vi "RealtimeDNITrack.vi"() -> ()   [LabVIEW 2017]
uses:
  <extravilib>/ChannelInstances/Tag-bool.lvlib
  <vilib>/platform/TimedLoop/XDataNode/XDataNode.xnode
  <vilib>/Platform/TimedLoop/XDataNode/nitl_modes.ctl
  <vilib>/Platform/TimedLoop/XDataNode/XDNodeRunTimeDep.lvlib
  <vilib>/Platform/TimedLoop/XDataNode/wakeup.ctl
  <vilib>/Platform/TimedLoop/XDataNode/timing_clust.ctl
  <vilib>/daq.io/MQTT LabVIEW Client/MQTT_Functions.lvlib
  <vilib>/daq.io/MQTT LabVIEW Client/Controls/MessageType.ctl
  <vilib>/daq.io/MQTT LabVIEW Client/Controls/Retain_Flag.ctl
  <vilib>/daq.io/MQTT LabVIEW Client/Controls/DUP_Flag.ctl
  <vilib>/daq.io/MQTT LabVIEW Client/Controls/QoS.ctl
  C:/Users/Labview/Downloads/Two Loops Ap/Two Loops Ap/Channel Scan Functional Global Op.ctl
  <vilib>/daq.io/MQTT LabVIEW Client/Controls/Connect_Flags.ctl
  <vilib>/daq.io/MQTT LabVIEW Client/Controls/Connection_Return_Codes.ctl
panel:
  in  "Tab Control":T1(tab)
  out "Corrected Phi":string
  out "Corrected Theta":string
  out "Current Time":string
  out "Corrected DNI":dbl
  in  "Working Directory":path=path "G:/Chad/Tracking Software/Analysis/LabVIEW-Outdoor-Tracking-App"
  out "Time of tracking start":string
  out "Sunset":string
  out "Sunrise":string
  in  "stop":bool
  in  "Stop Reading":bool
  out "standard error 3":string
  out "return code 3":i32
  in  "Script 3":string="solar_system.py"
  out "standard error":string
  out "return code":i32
  in  "error in (no error)":errorcluster
  in  "Sample Frequency (minutes)":string="1"
  out "Seconds to wait\nfor next minute":dbl
  in  "Script":string="cos_correct_v2.py"
  in  "Script 2":string="angle_to_position.py"
  out "standard error 2":string
  out "return code 2":i32
  out "Time":string
  out "Current Y":dbl
  out "Cos Corrected DNI":cluster{dbl[], dbl[]}(graph)
  out "Tracking":cluster{"X Coords":dbl[], "Y Coords":dbl[]}[](graph)
  out "Current X":dbl
  in  "Show full history":bool
  out "Waveform Graph":dbl[][](graph)
  in  "X Length":i32
  in  "Client ID":string="LVSubscribeClient"
  in  "Connect Flags":T2
  out "Granted QoS Levels":T3[](array[typedef])
  in  "Subscription Info Array":cluster{"Topic":string, "QoS":T3}[](array[cluster])=[{"Topic"="testtopic/LVMQTT", "QoS"=enum."At most once"}]
  in  "MQTT Broker":cluster{"address (IP)":string, "port":u16}={"address (IP)"="broker.hivemq.com", "port"=1883}
  out "Connection Status":T4=enum."Connection refused: Server unavailable"
  out "Messages":T6(array[cluster])
  out "MQTT Feed":string
  in  "Ping period (ms)":u32
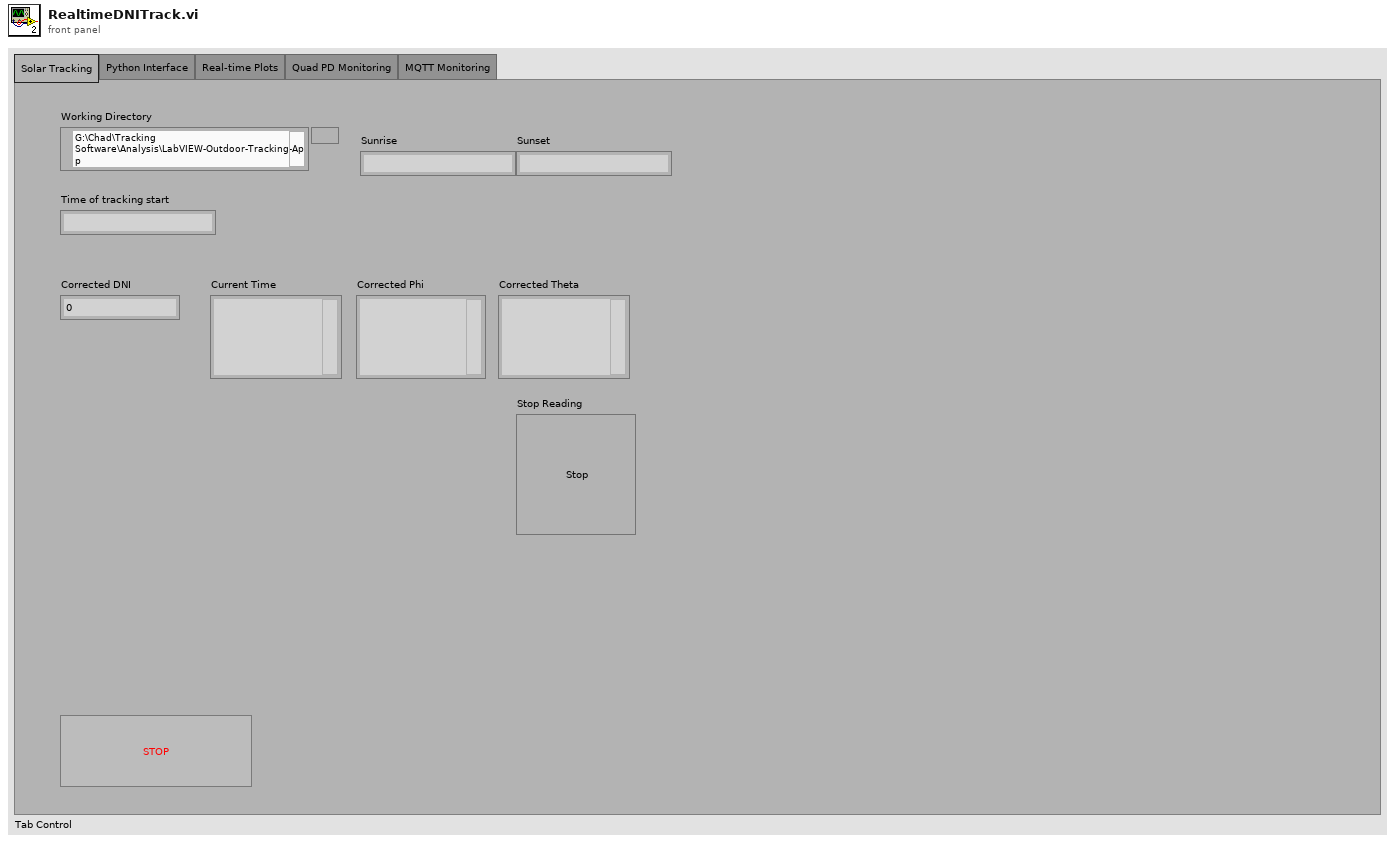
[diagram p1: front panel]
types:
  T1 = enum32{"Solar Tracking", "Python Interface", "Real-time Plots", "Quad PD Monitoring", "MQTT Monitoring"}
  T2 = typedef "MQTT_Functions.lvlib/Connect_Flags.ctl" = cluster{"user name":bool, "password":bool, "will retain":bool, "will flag":bool, "clean session":bool, "reserved":bool, "will QoS":T3}
  T3 = typedef "MQTT_Functions.lvlib/QoS.ctl" = enum8{"At most once", "At least once", "Exactly once", "Reserved"}
  T4 = typedef "MQTT_Functions.lvlib/Connection_Return_Codes.ctl" = enum16{"Connection accepted", "Connection refused: unacceptable protocol version", "Connection refused: identifier rejected", "Connection refused: Server unavailable", "Connection refused: bad user name or password", "Connection refused: not authorized"}
  T5 = typedef "MQTT_Functions.lvlib/MessageType.ctl" = enum32{"Reserved", "CONNECT", "CONNACK", "PUBLISH", "PUBACK", "PUBREC", "PUBREL", "PUBCOMP", "SUBSCRIBE", "SUBACK", "UNSUBSCRIBE", "UNSUBACK", "PINGREQ", "PINGRESP", "DISCONNECT", "Reserved2"}
  T6 = cluster{"Message ID":u16, "Topic Name":string, "Message ":string, "MessageType":T5}[]
  T7 = typedef "XDNodeRunTimeDep.lvlib/timing_clust.ctl" = cluster{"Expected End [f-1]":u64, "Actual End [f-1]":u64, "Finished Late? [f-1]":bool, "Expected End [i-1]":u64, "Actual End [i-1]":u64, "Finished Late? [i-1]":bool, "Expected Start [i]":u64, "Actual Start [i]":u64, "Expected Start [f]":u64, "Actual Start [f]":u64, "Source Name":string, "Structure Name":string, "Period":i64, "Deadline":i64, "Offset":i64, "Start":i64, "Priority":i32, "Timeout":i32, "Mode":T8, "Wakeup Reason":T9, "Error":errorcluster, "Source Type":string, "Secondary Source Type":string, "Global End Time":u64, "Global Start Time":u64, "Frame Duration":u64, "Iteration Duration":u64, "Assigned CPU":i32, "I/O Scan Engine Mode":u32}
  T8 = typedef "XDNodeRunTimeDep.lvlib/nitl_modes.ctl" = enum32{"No Change", "Process missed periods, maintain original phase", "Discard missed periods, maintain original phase", "Process missed periods, ignore original phase", "Discard missed periods, ignore original phase"}
  T9 = typedef "XDNodeRunTimeDep.lvlib/wakeup.ctl" = enum32{"Normal", "Aborted", "Asynchronous wakeup", "Timing source error", "Timed loop error", "Timeout"}
  T10 = typedef "MQTT_Functions.lvlib/DUP_Flag.ctl" = bool
  T11 = typedef "MQTT_Functions.lvlib/Retain_Flag.ctl" = bool
  T12 = cluster{"QoS":T3, "DUP":T10, "Retain":T11, "Keep Alive (sec)":u16}
  T13 = enum16{"None", "On Hover", "On Key Focus", "On Hover or Key Focus"}
  T14 = typedef "Channel Scan Functional Global Op.ctl" = enum16{"Init", "Insert Value", "Get Values"}
  T15 = cluster{"Message ID":u16, "Topic Name":string, "Message":string, "MessageType":T5}[]
  T16 = cluster{cluster{"X Coords":dbl[], "Y Coords":dbl[]}, cluster{dbl[], dbl[]}, cluster{dbl[], dbl[]}}
  T17 = cluster{"Message ID":u16, "Topic Name":string, "Message":string, "MessageType":T5}
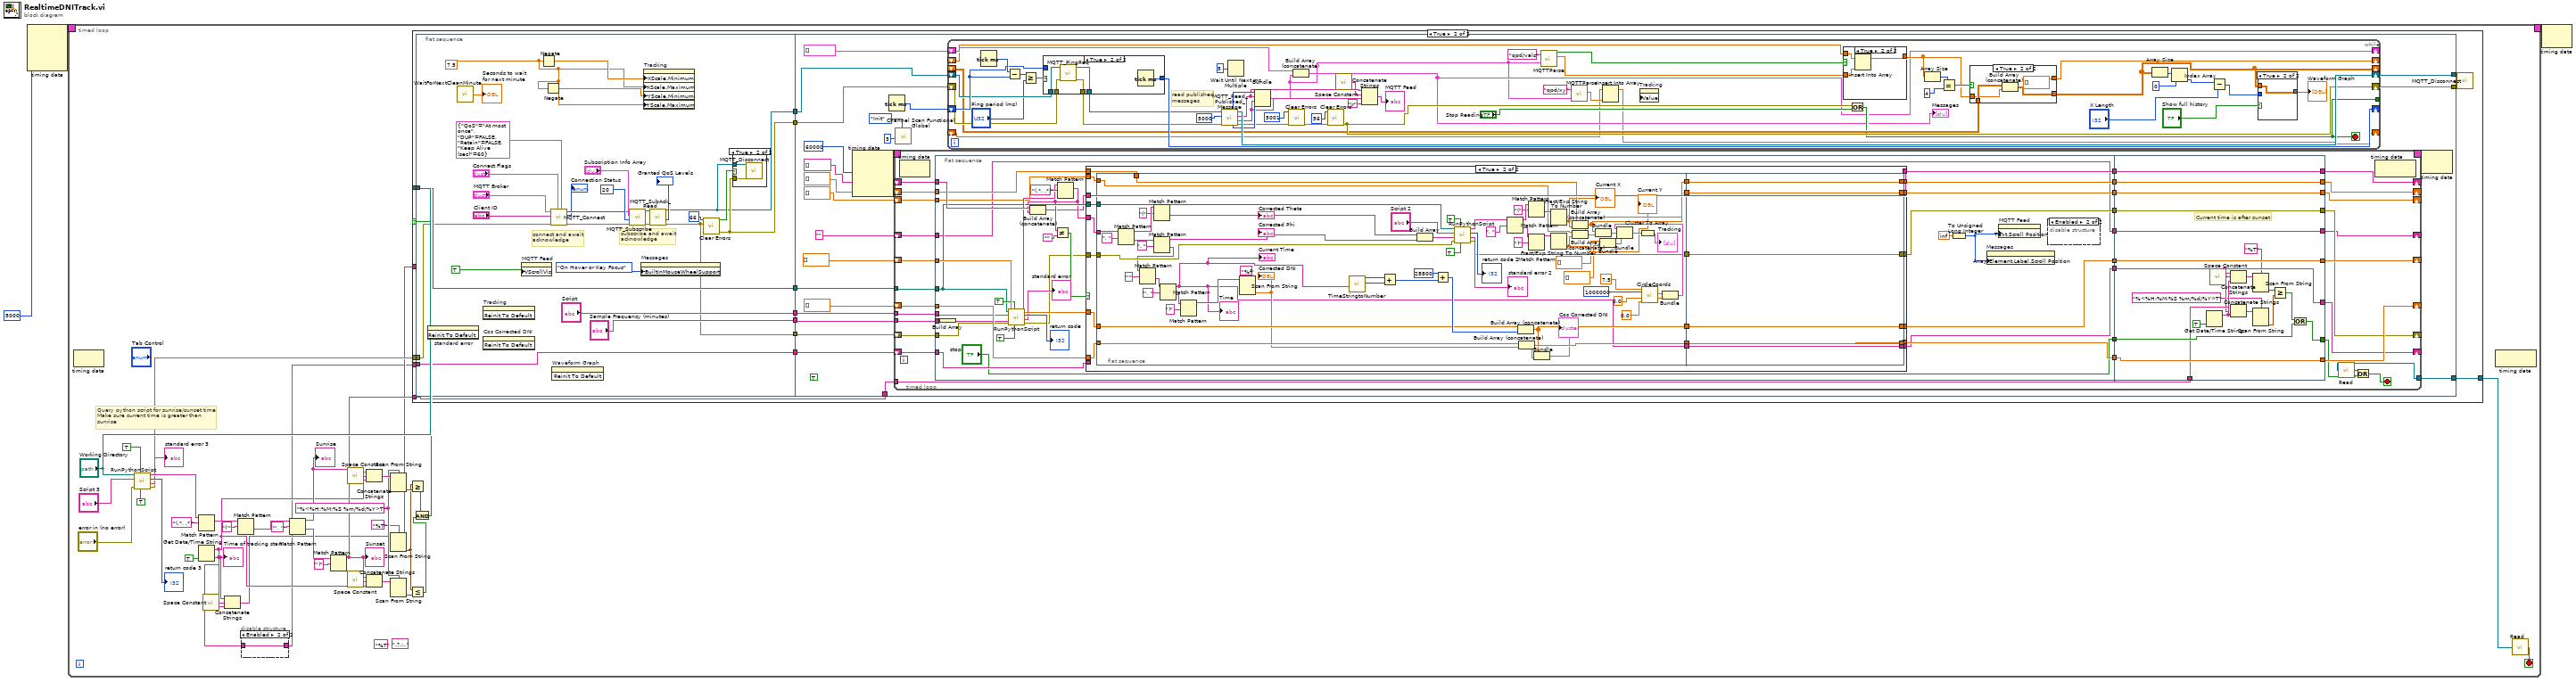
[diagram p0: block diagram]
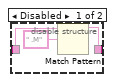
[diagram p2: hidden frame]
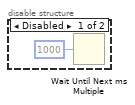
[diagram p5: hidden frame]
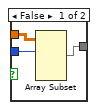
[diagram p7: hidden frame]
diagram:
  n1 = node-c288(i64 5000 ("Period")) -> (w3:T7)  [unwired: 3 in]
  n2 = timed-loop {
    timing: w3 -> [_]
    timing-out: [_] -> w2
    stop <- w41 stop-if-true
    w8 = "%<%H:%M:%S %m/%d/%Y>T" ("format string")
    (unwired) "%T" ("format string")
    (unwired) ".?.:.." ("regular expression")
    # "Query python script for sunrise/sunset time\nMake sure current time is greater than\nsunrise"
    n3 = node-c288() -> ()  [unwired: 1 in, 1 out]
    n4 = call "RunPythonScript.vi"("Run minimized? (F)"=TRUE, "Wait until completion? (T)"=TRUE, "error in (no error)"="error in (no error)", "Script"="Script 3", "Script Directory"="Working Directory") -> ("error out"=w23:errorcluster, "standard error"=→"standard error 3":string, "return code"=→"return code 3":i32, "standard output"=w37:string)  [unwired: 3 in]
    n5 = Match Pattern(string=w37, regular expression="(.*, .*)") -> (match substring=w36:string)  [unwired: 1 in, 3 out]
    n6 = Get Date/Time String(want seconds? (F)=TRUE) -> (date string=w14:string, time string=w5:string)  [unwired: 2 in]
    "Time of tracking start" <- w5
    n7 = call <vilib>:"Space Constant.vi"() -> ("String"=w22:string)
    n8 = Concatenate Strings(w5, w22, w14) -> (w6:string)
    n9 = Match Pattern(string=w36, regular expression="('") -> (after substring=w32:string)  [unwired: 1 in, 3 out]
    n10 = disable-structure shown="Enabled" {
      disable-tunnel: w5 -> [w44 w45]
      disable-tunnel: [w42 w45] -> w4
      frame Disabled {
        n11 = Match Pattern(string=w44, regular expression=" .M") -> (before substring=w42:string)  [unwired: 1 in, 3 out]
      }
      frame Enabled {
      }
    }
    n12 = Match Pattern(string=w32, regular expression="', '") -> (before substring=w19:string, after substring=w31:string)  [unwired: 1 in, 2 out]
    "Sunrise" <- w19
    n13 = Match Pattern(string=w31, regular expression="')") -> (before substring=w15:string)  [unwired: 1 in, 3 out]
    "Sunset" <- w15
    n14 = call <vilib>:"Space Constant.vi"() -> ("String"=w21:string)
    n15 = call <vilib>:"Space Constant.vi"() -> ("String"=w17:string)
    n16 = Concatenate Strings(w19, w21, w14) -> (w20:string)
    n17 = Concatenate Strings(w15, w17, w14) -> (w16:string)
    n18 = Scan From String(format string=w8, input string=w20) -> (output 1=w24:timestamp)  [unwired: 3 in, 3 out]
    n19 = Scan From String(format string="%T", input string=w6) -> (output 1=w18:timestamp)  [unwired: 3 in, 3 out]
    n20 = Scan From String(format string=w8, input string=w16) -> (output 1=w13:timestamp)  [unwired: 3 in, 3 out]
    n21 = Greater Or Equal?(x=w18, y=w24) -> (x >= y?=w12:bool)
    n22 = Less Or Equal?(x=w18, y=w13) -> (x <= y?=w11:bool)
    n23 = And(x=w12, y=w11) -> (x .and. y?=w10:bool)
    n24 = case shown="True" w10 {
      tunnel: "Working Directory" -> [_ w55]
      tunnel: w23 -> [_ w54]
      tunnel: w15 -> [_ w52]
      tunnel: [_ w53] -> w9
      tunnel: w6 -> [_ _]
      tunnel: w4 -> [_ w50]
      frame False {
      }
      frame True {
        n25 = flat-sequence {
          tunnel: [w64] -> w56
          tunnel: ["Script"] -> w57
          tunnel: [w82] -> w58
          tunnel: ["Sample Frequency (minutes)"] -> w59
          tunnel: w55 -> [w82]
          tunnel: w54 -> [w81]
          tunnel: w50 -> [w78]
          tunnel: [w78] -> w51
          tunnel: [w61] -> w49
          tunnel: [w60] -> w46
          tunnel: w59 -> [w106]
          tunnel: w58 -> [w107]
          tunnel: w57 -> [w108]
          tunnel: w56 -> [w102]
          tunnel: [w95] -> w53
          tunnel: w52 -> [w104]
          tunnel: w51 -> [w103]
          tunnel: w49 -> [w98]
          tunnel: [w96] -> w48
          tunnel: [w99] -> w47
          tunnel: w46 -> [w97]
          frame #0 {
            w85 = 7.5
            # "connect and await\nacknowledge"
            # "subscribe and await\nacknowledge"
            n26 = invoke on="standard error" class="Str" method="Reinit To Default"() -> ()  [unwired: 3 in, 3 out]
            n27 = call "WaitForNextCleanMinute.vi"() -> ("Seconds to wait"=→"Seconds to wait\nfor next minute":dbl)  [unwired: 1 in]
            n28 = invoke on="Tracking" class="XYGraph (strict)" method="Reinit To Default"() -> ()  [unwired: 3 in, 3 out]
            n29 = invoke on="Cos Corrected DNI" class="XYGraph (strict)" method="Reinit To Default"() -> ()  [unwired: 3 in, 3 out]
            n30 = property on="MQTT Feed" class="Str"("VScrollVis"=TRUE ("Vertical Scrollbar Visible")) -> ()  [unwired: 2 in, 2 out]
            n31 = Negate(x=w85) -> (-x=w87:dbl)
            n32 = Negate(x=w85) -> (-x=w86:dbl)
            n33 = call <vilib>:"MQTT_Connect.vi"("Connect Meta"=T12 {"QoS"=enum."At most once", "DUP"=FALSE, "Retain"=FALSE, "Keep Alive (sec)"=60}, "Client ID"="Client ID", "Connect Flags"="Connect Flags", "error in (no error)"=w81, "MQTT Broker"="MQTT Broker") -> ("error out"=w66:errorcluster, "Connection Status"=→"Connection Status":T4, "connection ID out"=w68:refnum<k5>)  [unwired: 4 in]
            n34 = invoke on="Waveform Graph" class="WFGraph (strict)" method="Reinit To Default"() -> ()  [unwired: 3 in, 3 out]
            n35 = call <vilib>:"MQTT_Subscribe.vi"("error in (no error)"=w66, "Message ID"=u16 20, "Subscription Info Array"="Subscription Info Array", "connection ID"=w68) -> ("error out"=w72:errorcluster, "connection ID out"=w73:refnum<k5>)  [unwired: 6 in]
            n36 = property on="Messages" class="Arr (strict)"("BuiltInMouseWheelSupport"=T13."On Hover or Key Focus" ("Built-In Mouse Wheel Support")) -> ()  [unwired: 2 in, 2 out]
            n37 = property on="Tracking" class="XYGraph (strict)"("XScale.Minimum"=w87, "XScale.Maximum"=w85, "YScale.Minimum"=w86, "YScale.Maximum"=w85) -> ()  [unwired: 2 in, 2 out]
            n38 = call <vilib>:"MQTT_SubAck_Read.vi"("error in (no error)"=w72, "connection ID"=w73) -> ("error out"=w64:errorcluster, "Granted QoS Levels"=→"Granted QoS Levels":T3[], "connection ID out"=w60:refnum<k5>)  [unwired: 7 in]
            n39 = call <vilib>:"Clear Errors.vi"("error in (no error)"=w64, "specific error code to clear (0: all)"=66) -> ("error out"=w61:errorcluster, "specific error cleared?"=w62:bool)  [unwired: 4 in]
            n40 = case shown="True" w62 {
              tunnel: w60 -> [_ w89]
              tunnel: w61 -> [_ w88]
              frame False {
              }
              frame True {
                n41 = call <vilib>:"MQTT_Disconnect.vi"("error in (no error)"=w88, "connection ID"=w89) -> ()  [unwired: 9 in, 1 out]
              }
            }
          }
          frame #1 {
            (unwired) TRUE ("Key Focus")
            n42 = node-c288(i64 60000 ("Period")) -> (w94:T7)  [unwired: 3 in]
            n43 = Tick Count (ms)() -> (millisecond timer value=w100:u32)
            n44 = timed-loop {
              tunnel: w106 -> [w141]
              shift-right: [w145] -> _
              shift-left: dbl[] [] -> [w146]
              shift-right: [w144] -> _
              shift-left: dbl[] [] -> [w142]
              shift-right: [w134] -> _
              shift-left: string[] [] -> [w143]
              tunnel: w107 -> [w135]
              tunnel: w108 -> [w140]
              shift-right: [w138] -> _
              shift-left: dbl[] [] -> [w137]
              shift-right: [w136] -> _
              shift-left: dbl[] [] -> [w139]
              shift-right: [w126] -> _
              shift-left: w103 -> [w125]
              tunnel: w104 -> [w124]
              tunnel: [w117] -> w95
              shift-right: [w121] -> _
              shift-left: "" -> [w120]
              shift-right: [w123] -> _
              shift-left: w102 -> [w119]
              timing: w94 -> [_]
              timing-out: [_] -> w93
              stop <- w114 stop-if-true
              n45 = node-c288() -> ()  [unwired: 1 in, 1 out]
              n46 = flat-sequence {
                tunnel: w146 -> [w180]
                tunnel: w143 -> [w177]
                tunnel: w142 -> [w176]
                tunnel: w119 -> [w175]
                tunnel: w141 -> [w170]
                tunnel: w140 -> [w168]
                tunnel: w139 -> [w167]
                tunnel: w137 -> [w165]
                tunnel: w135 -> [w163]
                tunnel: [w179] -> w133
                tunnel: [w178] -> w132
                tunnel: [w166] -> w131
                tunnel: ["stop"] -> w130
                tunnel: [w164] -> w129
                tunnel: [w150] -> w128
                tunnel: [w157] -> w127
                tunnel: w125 -> [w156]
                tunnel: [w151] -> w122
                tunnel: w120 -> [w149]
                tunnel: [w149] -> w118
                tunnel: [w296] -> w134
                tunnel: [w297] -> w136
                tunnel: [w298] -> w138
                tunnel: [w299] -> w144
                tunnel: [w300] -> w145
                tunnel: w133 -> [w300]
                tunnel: w132 -> [w299]
                tunnel: w131 -> [w298]
                tunnel: w130 -> [w295]
                tunnel: w129 -> [w297]
                tunnel: w128 -> [w296]
                tunnel: w127 -> [w290]
                tunnel: [w290] -> w126
                tunnel: w124 -> [w288]
                tunnel: [w283] -> w116
                tunnel: [w282] -> w123
                tunnel: w122 -> [w282]
                tunnel: [w281] -> w121
                tunnel: w118 -> [w281]
                frame #0 {
                  n47 = Build Array(w170) -> (w169:string[])
                  n48 = call "RunPythonScript.vi"("Run minimized? (F)"=TRUE ("run minimized? (F)"), "Wait until completion? (T)"=TRUE ("wait until completion? (T)"), "error in (no error)"=w175, "Array of arguments to script"=w169, "Script"=w168, "Script Directory"=w163) -> ("error out"=w152:errorcluster, "standard error"=→"standard error":string, "return code"=→"return code":i32, "standard output"=w172:string)  [unwired: 2 in]
                  n49 = Match Pattern(string=w172, regular expression="(.*, .*)") -> (match substring=w160:string)  [unwired: 1 in, 3 out]
                  n50 = Build Array (concatenate)(w177, w160) -> (w158:string[])
                  n51 = Not Equal?(x=w160, y="") -> (x != y?=w159:bool)
                  n52 = case shown="True" w159 {
                    tunnel: w180 -> [w186 w209]
                    tunnel: [w186 w208] -> w179
                    tunnel: [w187 w207] -> w178
                    tunnel: w176 -> [w187 w206]
                    tunnel: w167 -> [w189 w205]
                    tunnel: [w188 w204] -> w166
                    tunnel: w165 -> [w188 w203]
                    tunnel: [w189 w202] -> w164
                    tunnel: w163 -> [_ w201]
                    tunnel: w160 -> [_ w198]
                    tunnel: [w185 w190] -> w150
                    tunnel: w158 -> [w185 w190]
                    tunnel: [w184 w197] -> w157
                    tunnel: w156 -> [w184 _]
                    tunnel: w152 -> [w183 w200]
                    tunnel: [w183 w199] -> w151
                    frame False {
                    }
                    frame True {
                      n53 = flat-sequence {
                        tunnel: w209 -> [w273]
                        tunnel: w206 -> [w265]
                        tunnel: w205 -> [w252]
                        tunnel: w203 -> [w248]
                        tunnel: w201 -> [w235]
                        tunnel: w200 -> [w232]
                        tunnel: w198 -> [w223]
                        tunnel: [w272] -> w196
                        tunnel: [w271] -> w195
                        tunnel: [w251] -> w194
                        tunnel: [w243] -> w193
                        tunnel: [w231] -> w192
                        tunnel: [w213] -> w191
                        tunnel: [w274] -> w197
                        tunnel: [w275] -> w199
                        tunnel: [w276] -> w202
                        tunnel: [w277] -> w204
                        tunnel: [w278] -> w207
                        tunnel: [w279] -> w208
                        tunnel: w196 -> [w279]
                        tunnel: w195 -> [w278]
                        tunnel: w194 -> [w277]
                        tunnel: w193 -> [w276]
                        tunnel: w192 -> [w275]
                        tunnel: w191 -> [w274]
                        frame #0 {
                          n54 = Match Pattern(string=w223, regular expression=", ") -> (before substring=w226:string, after substring=w227:string)  [unwired: 1 in, 2 out]
                          n55 = Match Pattern(string=w226, regular expression="(") -> (after substring=w221:string)  [unwired: 1 in, 3 out]
                          "Corrected Theta" <- w221
                          n56 = Match Pattern(string=w227, regular expression=", ") -> (before substring=w220:string, after substring=w217:string)  [unwired: 1 in, 2 out]
                          "Corrected Phi" <- w220
                          n57 = Match Pattern(string=w217, regular expression="'") -> (after substring=w215:string)  [unwired: 1 in, 3 out]
                          n58 = Match Pattern(string=w215, regular expression="', ") -> (before substring=w213:string, after substring=w214:string)  [unwired: 1 in, 2 out]
                          "Current Time" <- w213
                          "Time" <- w213
                          n59 = Match Pattern(string=w214, regular expression=")") -> (before substring=w219:string)  [unwired: 1 in, 3 out]
                          n60 = Scan From String(format string="%f", input string=w219) -> (output 1=w229:dbl)  [unwired: 3 in, 3 out]
                          "Corrected DNI" <- w229
                          n61 = call "TimeStringtoNumber.vi"("time string"=w213) -> ("Minutes"=w269:i32, "Hours"=w270:i32)  [unwired: 3 out]
                          n62 = Add(x=w270, y=w269) -> (x+y=w268:i32)
                          n63 = Build Array(w221, w220) -> (w262:string[])
                          n64 = Add(x=28800, y=w268) -> (x+y=w266:i32)
                          n65 = call "RunPythonScript.vi"("Run minimized? (F)"=TRUE ("run minimized? (F)"), "Wait until completion? (T)"=TRUE ("wait until completion? (T)"), "error in (no error)"=w232, "Array of arguments to script"=w262, "Script"="Script 2", "Script Directory"=w235) -> ("error out"=w231:errorcluster, "standard error"=→"standard error 2":string, "return code"=→"return code 2":i32, "standard output"=w260:string)  [unwired: 2 in]
                          n66 = Match Pattern(string=w260, regular expression=", ") -> (before substring=w257:string, after substring=w258:string)  [unwired: 1 in, 2 out]
                          n67 = Build Array (concatenate)(w265, w266) -> (w271:dbl[])
                          n68 = Build Array (concatenate)(w273, w229) -> (w272:dbl[])
                          n69 = Match Pattern(string=w257, regular expression="(") -> (after substring=w254:string)  [unwired: 1 in, 3 out]
                          n70 = Match Pattern(string=w258, regular expression=")") -> (before substring=w253:string)  [unwired: 1 in, 3 out]
                          n71 = Bundle(w271, w272) -> (→"Cos Corrected DNI":cluster{dbl[], dbl[]})  [unwired: 1 in]
                          n72 = Fract/Exp String To Number(string=w254) -> (number=w237:dbl)  [unwired: 3 in, 1 out]
                          "Current X" <- w237
                          n73 = Fract/Exp String To Number(string=w253) -> (number=w236:dbl)  [unwired: 3 in, 1 out]
                          "Current Y" <- w236
                          n74 = Build Array (concatenate)(w248, w237) -> (w251:dbl[])
                          n75 = Build Array (concatenate)(w252, w236) -> (w243:dbl[])
                          n76 = Bundle(w251, w243) -> (w238:cluster{dbl[], dbl[]})  [unwired: 1 in]
                          n77 = Bundle(dbl[] [], dbl[] []) -> (w212:cluster{dbl[], dbl[]})  [unwired: 1 in]
                          n78 = call "CircleCoords.vi"("Magnitude"=7.5, "Number of Points"=1000000, "X Origin"=0.0, "Y Origin"=0.0) -> ("X Coords"=w242:dbl[], "Y Coords"=w241:dbl[])  [unwired: 1 in]
                          n79 = Bundle("X Coords"=w242, "Y Coords"=w241) -> (w239:cluster{"X Coords":dbl[], "Y Coords":dbl[]})  [unwired: 1 in]
                          n80 = Bundle(w239, w238, w212) -> (w240:T16)  [unwired: 1 in]
                          n81 = Cluster To Array(cluster=w240) -> (array=→"Tracking":cluster{"X Coords":dbl[], "Y Coords":dbl[]}[])
                        }
                        frame #1 {
                        }
                      }
                    }
                  }
                  n82 = To Unsigned Long Integer(number=inf) -> (unsigned 32bit integer=w154:u32)
                  n83 = property on="Messages" class="Arr (strict)"("Array Element.Label.Scroll Position"=w154) -> ()  [unwired: 2 in, 2 out]
                  n84 = property on="MQTT Feed" class="Str"("Text.Scroll Position"=w154) -> ()  [unwired: 2 in, 2 out]
                  n85 = disable-structure shown="Enabled" {
                    frame Disabled {
                      n86 = Wait Until Next ms Multiple(millisecond multiple=u32 1000) -> ()  [unwired: 1 out]
                    }
                    frame Enabled {
                    }
                  }
                }
                frame #1 {
                  # "Current time is after sunset"
                  n87 = Get Date/Time String(want seconds? (F)=TRUE) -> (date string=w289:string)  [unwired: 2 in, 1 out]
                  n88 = call <vilib>:"Space Constant.vi"() -> ("String"=w287:string)
                  n89 = Concatenate Strings(w290, w287, w289) -> (w286:string)
                  n90 = Concatenate Strings(w288, w287, w289) -> (w285:string)
                  n91 = Scan From String(format string="%T", input string=w286) -> (output 1=w293:timestamp)  [unwired: 3 in, 3 out]
                  n92 = Scan From String(format string="%<%H:%M:%S %m/%d/%Y>T", input string=w285) -> (output 1=w292:timestamp)  [unwired: 3 in, 3 out]
                  n93 = Greater Or Equal?(x=w293, y=w292) -> (x >= y?=w294:bool)
                  n94 = Or(x=w294, y=w295) -> (x .or. y?=w283:bool)
                }
              }
              n95 = call <extravilib>:"Read.vi"("channel"=w117) -> ("element"=w115:bool)  [unwired: 1 in, 1 out]
              n96 = Or(x=w115, y=w116) -> (x .or. y?=w114:bool)
              n97 = node-c288() -> ()  [unwired: 1 in, 1 out]
            }
            n98 = call "Channel Scan Functional Global.vi"("Operation"=Channel_Scan_Functional_Global_Op."Init", "Scan List Size"=3) -> ()  [unwired: 9 in, 1 out]
            n99 = while {
              shift-right: [w312] -> _
              shift-left: T15 [] ("Array") -> [w346]
              shift-right: [w335] -> w96
              shift-left: w98 -> [w348]
              shift-right: [w343] -> w99
              shift-left: w97 -> [w349]
              shift-right: [w354] -> _
              shift-left: w100 -> [w350]
              shift-right: [w329] -> _
              shift-left: _ -> [w334]
              shift-right: [w324] -> _
              shift-left: _ -> [w328]
              tunnel: [w318] -> _
              shift-right: [w305] -> _
              shift-left: _ -> [w306]
              stop <- w318 stop-if-true
              # "read published\nmessages"
              n100 = Tick Count (ms)() -> (millisecond timer value=w353:u32)
              n101 = Subtract(x=w353, y=w350) -> (x-y=w351:u32)
              n102 = Greater Or Equal?(x=w351, y="Ping period (ms)") -> (x >= y?=w352:bool)
              n103 = case shown="True" w352 {
                tunnel: [w373 w378] -> w354
                tunnel: w350 -> [w373 _]
                tunnel: w348 -> [w371 w377]
                tunnel: w349 -> [w372 w376]
                tunnel: [w371 w375] -> w344
                tunnel: [w372 w374] -> w345
                frame False {
                }
                frame True {
                  n104 = call <vilib>:"MQTT_PingReq.vi"("error in (no error)"=w377, "connection ID"=w376) -> ("error out"=w375:errorcluster, "connection ID out"=w374:refnum<k5>)  [unwired: 7 in, 1 out]
                  n105 = Tick Count (ms)() -> (millisecond timer value=w378:u32)
                }
              }
              n106 = call <vilib>:"MQTT_Read_Published_Message.vi"("error in (no error)"=w344, "timeout ms (25000)"=5000, "connection ID"=w345) -> ("error out"=w339:errorcluster, "Message"=w314:string, "Topic Name"=w316:string, "connection ID out"=w343:refnum<k5>, "MessageType"=w341:T5, "Message ID"=w342:u16)  [unwired: 3 in]
              n107 = Wait Until Next ms Multiple(millisecond multiple=u32 5) -> ()  [unwired: 1 out]
              n108 = Bundle("Message ID"=w342, "Topic Name"=w316, "Message"=w314, "MessageType"=w341) -> (w308:T17)  [unwired: 1 in]
              n109 = call <vilib>:"Clear Errors.vi"("error in (no error)"=w339, "specific error code to clear (0: all)"=5001) -> ("error out"=w336:errorcluster)  [unwired: 4 in, 1 out]
              n110 = Build Array (concatenate)(w346, w308) -> (w312:T15)
              "Messages" <- w312
              n111 = call <vilib>:"Clear Errors.vi"("error in (no error)"=w336, "specific error code to clear (0: all)"=56) -> ("error out"=w335:errorcluster)  [unwired: 4 in, 1 out]
              n112 = call <vilib>:"Space Constant.vi"() -> ("String"=w315:string)
              n113 = Concatenate Strings(w316, w315, w314, "\r") -> (→"MQTT Feed":string)
              n114 = call "MQTTParse.vi"("topic"="qpd/vals", "Input message"=w308) -> ("Success?"=w326:bool, "Double"=w327:dbl)  [unwired: 3 in, 1 out]
              n115 = call "MQTTParse.vi"("topic"="qpd/xy", "Input message"=w308) -> ("Double"=w307:dbl)  [unwired: 3 in, 2 out]
              n116 = Insert Into Array(array=w306, new element=w307) -> (w305:dbl[])  [unwired: 1 in]
              n117 = property on="Tracking" class="XYGraph (strict)" props=["Value"]() -> ()  [unwired: 3 in, 2 out]
              n118 = case shown="True" w326 {
                tunnel: w327 -> [_ w370]
                tunnel: [w367 w368] -> w330
                tunnel: w334 -> [w367 w369]
                frame False {
                }
                frame True {
                  n119 = Insert Into Array(array=w369, new element=w370) -> (w368:dbl[])  [unwired: 1 in]
                }
              }
              n120 = Or(x=w335, y="Stop Reading") -> (x .or. y?=w318:bool)
              n121 = Array Size(array=w330) -> (size(s)=w332:i32)
              n122 = Equal?(x=w332, y=4) -> (x = y?=w331:bool)
              n123 = case shown="True" w331 {
                tunnel: w330 -> [w362 w363]
                tunnel: [w362 dbl[] []] -> w329
                tunnel: [w361 w365] -> w324
                tunnel: w328 -> [w361 w364]
                frame False {
                }
                frame True {
                  n124 = Build Array (concatenate)(w364, w363) -> (w365:dbl[][])
                }
              }
              n125 = Array Size(array=w324) -> (size(s)=w322:i32[])
              n126 = Index Array(array=w322, index=0) -> (element=w320:i32)
              n127 = Subtract(x=w320, y="X Length") -> (x-y=w319:i32)
              n128 = case shown="True" "Show full history" {
                tunnel: [w359 w360] -> w325
                tunnel: w324 -> [w358 w360]
                tunnel: w319 -> [w357 _]
                frame False {
                  n129 = Array Subset(array=w358, index (row)=w357) -> (w359:dbl[][])  [unwired: 3 in]
                }
                frame True {
                }
              }
              "Waveform Graph" <- w325
            }
            n130 = node-c288(w93) -> ()  [unwired: 1 out]
          }
        }
        n131 = call <vilib>:"MQTT_Disconnect.vi"("error in (no error)"=w48, "connection ID"=w47) -> ()  [unwired: 9 in, 1 out]
      }
    }
    n132 = node-c288() -> ()  [unwired: 1 in, 1 out]
    n133 = call <extravilib>:"Read.vi"("channel"=w9) -> ("element"=w41:bool)  [unwired: 1 in, 1 out]
  }
  n134 = node-c288(w2) -> ()  [unwired: 1 out]
